vi "Write.ProcessData.vi"(8 "error in (no error)":errorcluster, 9 "Offset":i32, 10 "Values":dbl[](array[numeric]), 11 "Write in":refnum<class "Write.lvclass">) -> (0 "error out":errorcluster, 3 "Write out":refnum<class "Write.lvclass">)   [LabVIEW 2015, in "Data Access Engine.lvlib" / "Write.lvclass"]
uses:
  Write.lvclass
  Write.lvclass/Write.ctl
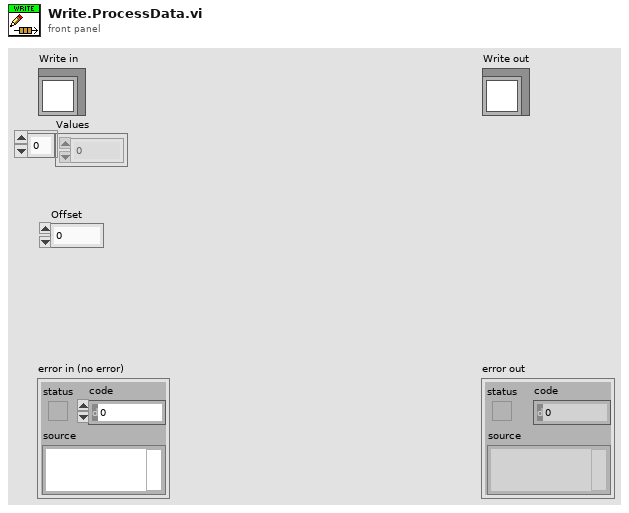
[diagram p1: front panel]
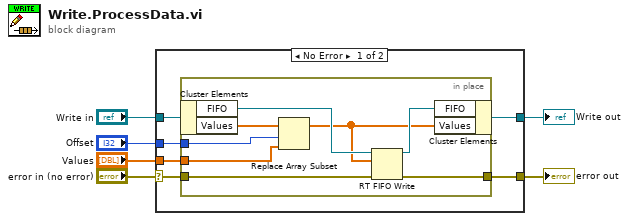
[diagram p0: block diagram]
diagram:
  n1 = case shown="No Error" "error in (no error)" {
    selector: "error in (no error)" -> [w9 w22]
    tunnel: [w8 w22] -> w5
    tunnel: [w11 w21] -> w3
    tunnel: "Write in" -> [w12 w21]
    tunnel: "Values" -> [w10 _]
    tunnel: "Offset" -> [w7 _]
    frame No Error {
      n2 = in-place {
        in-place-border: w10 -> [w16]
        in-place-border: w9 -> [w18]
        in-place-border: [w17] -> w8
        in-place-border: w7 -> [w13]
        n3 = in-place-cluster #1(w12) -> ("FIFO"=w20:refnum<k33>, "Values"=w15:dbl[])
        n4 = Replace Array Subset(array=w15, new element=w16, index=w13) -> (w14:dbl[])
        n5 = RT FIFO Write(0:w20, 1:w14, 3:w18) -> (8:w19:refnum<k33>, 11:w17:errorcluster)  [unwired: 2 in, 2 out]
        n6 = in-place-cluster #1("FIFO"=w19, "Values"=w14) -> (w11:refnum<class "Write.lvclass">)
      }
    }
    frame Error {
    }
  }
  "error out" <- w5
  "Write out" <- w3
